vi "Input_VI.vi"(8 "error in":errorcluster, 9 "Enable":bool=TRUE, 10 "input string":string, 11 "Text.Text Colors:BG Color":u32(colorbox)=16448250) -> (0 "error out":errorcluster, 1 "Boolean":bool, 2 "Continue 2":bool, 3 "Varaint out":string)   [LabVIEW 2021]
panel:
  in  "Variant name":string
  in  "OK":bool caption="Enter to continue"
  out "String":string
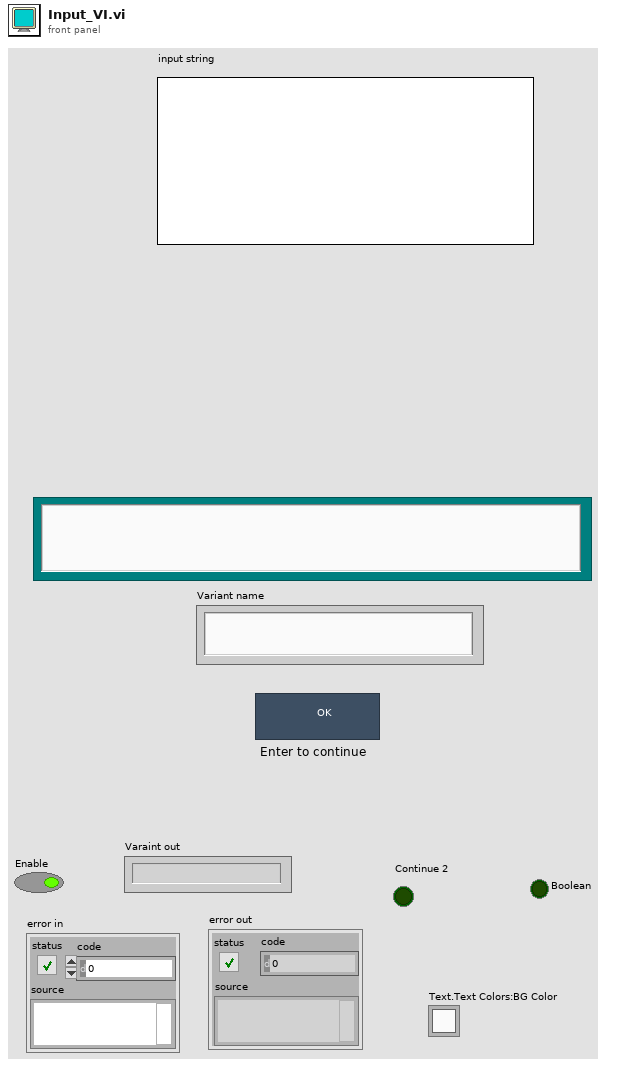
[diagram p1: front panel]
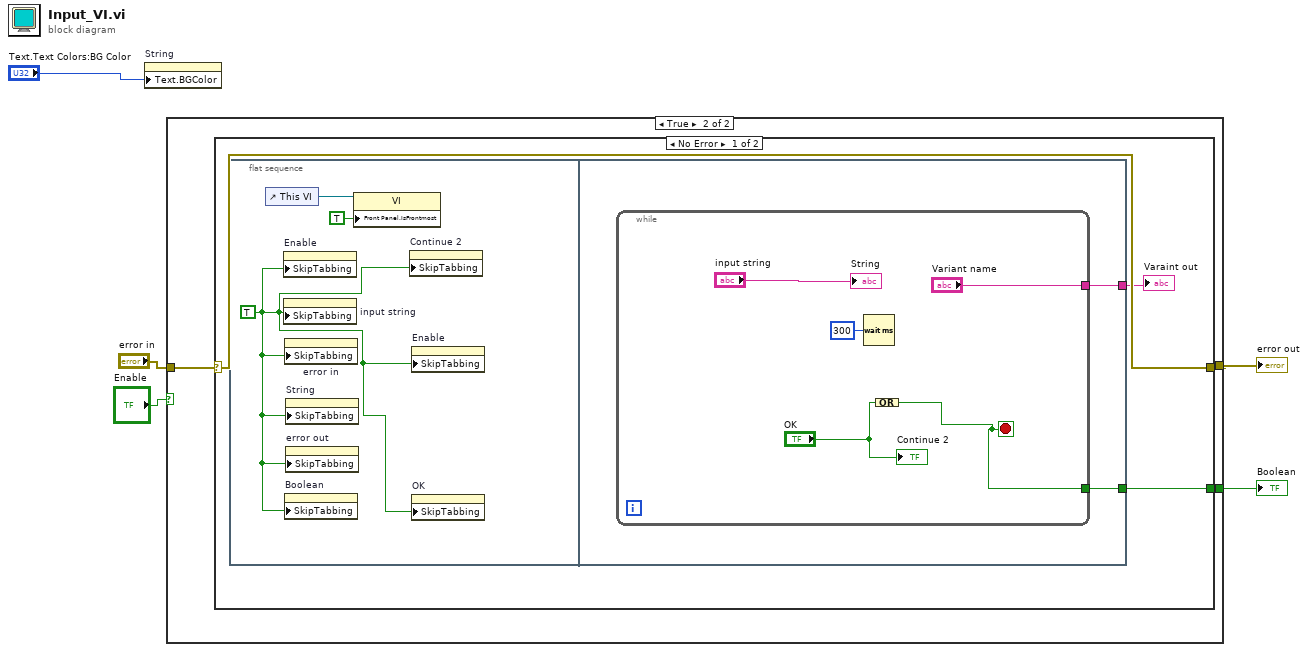
[diagram p0: block diagram]
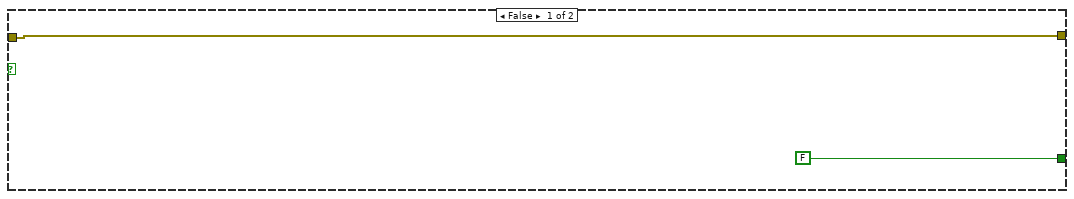
[diagram p2: hidden frame]
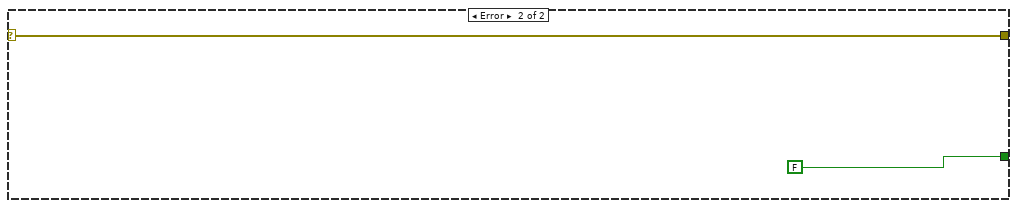
[diagram p3: hidden frame]
diagram:
  n1 = property on="String" class="Str"("Text.BGColor"="Text.Text Colors:BG Color") -> ()  [unwired: 2 in, 2 out]
  n2 = case shown="True" "Enable" {
    tunnel: "error in" -> [w7 w10]
    tunnel: [w7 w9] -> w4
    tunnel: [FALSE ("OK Button") w8] -> w2
    frame False {
    }
    frame True {
      n3 = case shown="No Error" w10 {
        selector: w10 -> [w13 w25]
        tunnel: [w13 w25] -> w9
        tunnel: [w12 FALSE ("OK Button")] -> w8
        frame No Error {
          n4 = flat-sequence {
            tunnel: [w18] -> w12
            tunnel: [w17] -> w11
            frame #0 {
              w14 = TRUE ("Skip When Tabbing")
              n5 = control-ref of="This VI"() -> (w16:refnum<vi>)
              n6 = property on="Enable" class="Bool (strict)"("SkipTabbing"=w14) -> ()  [unwired: 2 in, 2 out]
              n7 = property on="input string" class="Str"("SkipTabbing"=w14) -> ()  [unwired: 2 in, 2 out]
              n8 = property on="error in" class="Clust (strict)"("SkipTabbing"=w14) -> ()  [unwired: 2 in, 2 out]
              n9 = property on="Boolean" class="Bool (strict)"("SkipTabbing"=w14) -> ()  [unwired: 2 in, 2 out]
              n10 = property on="String" class="Str"("SkipTabbing"=w14) -> ()  [unwired: 2 in, 2 out]
              n11 = property on="error out" class="Clust (strict)"("SkipTabbing"=w14) -> ()  [unwired: 2 in, 2 out]
              n12 = property class="VI"(reference=w16, "Front Panel.IsFrontmost"=TRUE ("Front Panel Window:Is Frontmost")) -> ()  [unwired: 1 in, 2 out]
              n13 = property on="Continue 2" class="Bool"("SkipTabbing"=w14) -> ()  [unwired: 2 in, 2 out]
              n14 = property on="Enable" class="Bool (strict)"("SkipTabbing"=w14) -> ()  [unwired: 2 in, 2 out]
              n15 = property on="OK" class="Bool"("SkipTabbing"=w14) -> ()  [unwired: 2 in, 2 out]
            }
            frame #1 {
              n16 = while {
                tunnel: [w20] -> w18
                tunnel: ["Variant name"] -> w17
                stop <- w20 stop-if-true
                n17 = Wait (ms)(milliseconds to wait=u32 300) -> ()  [unwired: 1 out]
                n18 = Compound Arithmetic op=OR("OK") -> (w20:bool)
                "String" <- "input string"
                "Continue 2" <- "OK"
              }
            }
          }
          "Varaint out" <- w11
        }
        frame Error {
        }
      }
    }
  }
  "error out" <- w4
  "Boolean" <- w2
